vi "Report Iterations End.vi"(8 "error in":errorcluster, 9 "Iterator Error":errorcluster, 10 "Caller Enqueuer in":refnum<class "Message Enqueuer.lvclass">, 11 "Iterator Actor in":refnum<class "Abstract Iterator Actor.lvclass">) -> (0 "error out":errorcluster, 3 "Iterator Actor out":refnum<class "Abstract Iterator Actor.lvclass">)   [LabVIEW 2021, in "Iterator Actor.lvlib" / "Abstract Iterator Actor.lvclass"]
uses:
  Abstract Iterator Actor.lvclass
  <vilib>/ActorFramework/Message Enqueuer/Message Enqueuer.lvclass
  Abstract Iterator Actor.lvclass/Abstract Iterator Actor.ctl
  Iterator Actor/Iterator Actor Abstract Messages/Iterator Report Iterations End Msg/Iterator Report Iterations End Msg.lvclass
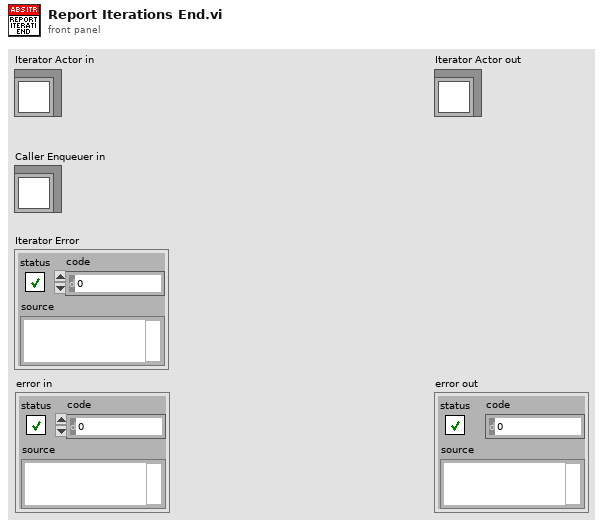
[diagram p1: front panel]
types:
  T1 = typedef "Iterator Actor.lvlib/Abstract Iterator Actor.lvclass/Stop Reason.ctl" = enum16{"Number of Iterations", "Time Elapsed", "Stopped Internally", "Stopped Externally"}
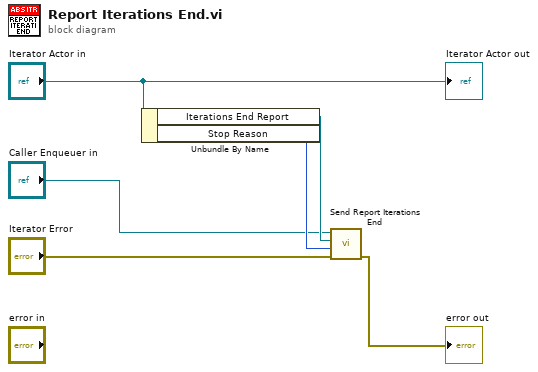
[diagram p0: block diagram]
diagram:
  n1 = Unbundle By Name("Iterator Actor in") -> ("Iterations End Report"=w4:refnum<class "Iterator Report Iterations End Msg.lvclass">, "Stop Reason"=w5:T1)
  n2 = call "Send Report Iterations End.vi"("error in (no error)"="Iterator Error", "Stop Reason"=w5, "Caller Error Handler"=w4, "Caller Enqueuer in"="Caller Enqueuer in") -> ("error out"=→"error out":errorcluster)  [unwired: 6 in, 1 out]
  "Iterator Actor out" <- "Iterator Actor in"
